vi "Init Command.vi"(5 "Sequencer":refnum<class "MessageQ.lvclass">, 6 "Variables":refnum<class "Variables.lvclass">, 7 "VolatusAPI":refnum<class "VolatusAPI.lvclass">, 8 "error in (no error)":refnum<class "MultiErrors.lvclass">, 10 "Command Config":refnum<class "Command Config.lvclass">, 11 "Reset Var Command in":refnum<class "Reset Var Command.lvclass">) -> (0 "error out":refnum<class "MultiErrors.lvclass">, 3 "Command":T1)   [LabVIEW 2020, in "VolatusSeq.lvlib" / "Reset Var Command.lvclass"]
uses:
  Reset Var Command.lvclass
  Reset Var Command.lvclass/Reset Var Command.ctl
  VolatusSeqConfig/Reset Var Command Config/Reset Var Command Config.lvclass
  VolatusSeqConfig/Command Type.ctl
  VolatusSeqConfig/VolatusSeqConfig.lvlib
  Volatus/MessageQ/MessageQ.lvclass
  messages/CmdDigital/Data.ctl
  messages/CmdDigital/CmdDigital.lvlib
  messages/CmdAnalog/Data.ctl
  messages/CmdAnalog/CmdAnalog.lvlib
  Send Type.ctl
  VolatusSeq.lvlib
  Command.ctl
  Variables/Variables.lvclass
  VolatusErrorUtilities/MultiErrors/MultiErrors.lvclass
  Volatus/VolatusAPI/VolatusAPI.lvclass
  VolatusSeqConfig/Command Config/Command Config.lvclass
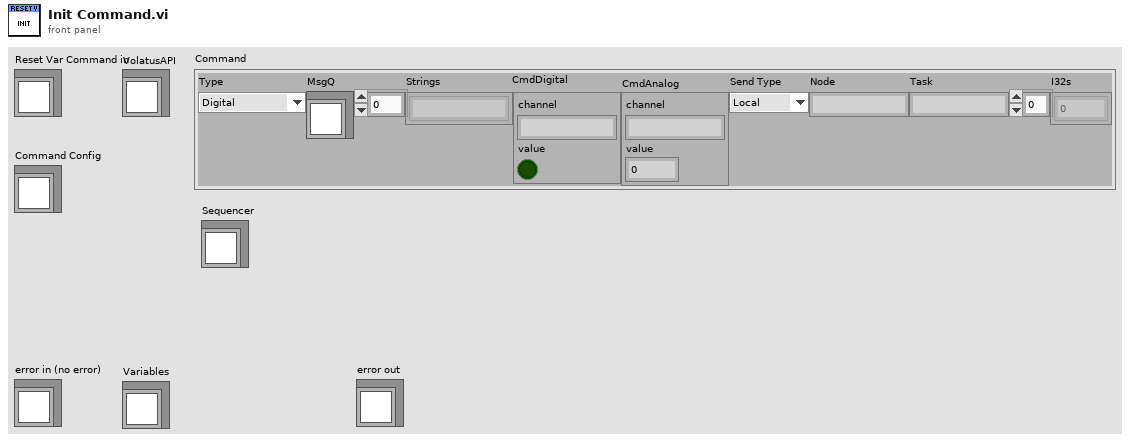
[diagram p1: front panel]
types:
  T1 = typedef "VolatusSeq.lvlib/Command.ctl" = cluster{"Type":T2, "MsgQ":refnum<class "MessageQ.lvclass">, "Strings":string[], "CmdDigital":T3, "CmdAnalog":T4, "Send Type":T5, "Node":string, "Task":string, "I32s":i32[]}
  T2 = typedef "VolatusSeqConfig.lvlib/Command Type.ctl" = enum16{"Digital", "Numeric", "Transition", "Stop", "StartLog", "StopLog", "Start", "Event", "Error", "HTTP", "ResetVar", "IncVar", "DecVar", "SaveVar", "LoadVar", "AddVar", "SubVar"}
  T3 = typedef "CmdDigital.lvlib/Data.ctl" = cluster{"channel":string, "value":bool}
  T4 = typedef "CmdAnalog.lvlib/Data.ctl" = cluster{"channel":string, "value":dbl}
  T5 = typedef "VolatusSeq.lvlib/Send Type.ctl" = enum16{"Local", "Remote"}
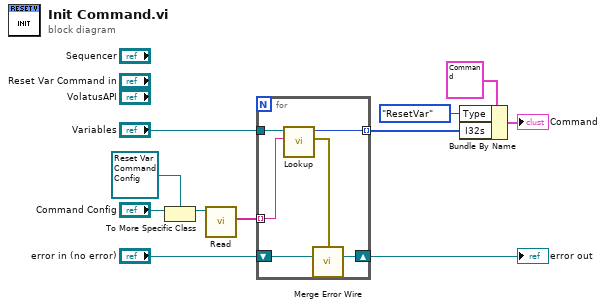
[diagram p0: block diagram]
diagram:
  n1 = To More Specific Class(target class=refnum<class "Reset Var Command Config.lvclass"> refnum ("VolatusSeqConfig.lvlib:Reset Var Command Config.lvclass"), reference="Command Config") -> (specific class reference=w9:refnum<class "Reset Var Command Config.lvclass">)  [unwired: 1 in, 1 out]
  n2 = call "Read.vi"("Reset Var Command Config in"=w9) -> ("Names"=w4:string[])  [unwired: 8 in, 2 out]
  n3 = for {
    shift-right: [w13] -> w5
    shift-left: "error in (no error)" -> [w14]
    tunnel: w4 -> [w16] mode=indexing
    tunnel: "Variables" -> [w17]
    tunnel: [w15] -> w2 mode=indexing
    n4 = call "Lookup.vi"("Name"=w16, "Variables in"=w17) -> ("error out"=w12:errorcluster, "Index"=w15:i32)  [unwired: 8 in]
    n5 = call "Merge Error Wire.vi"("error in (no error)"=w12, "MultiErrors in"=w14) -> ("MultiErrors out"=w13:refnum<class "MultiErrors.lvclass">)  [unwired: 13 in]
  }
  "error out" <- w5
  n6 = Bundle By Name(cluster=T1 {"Type"=enum."Digital", "MsgQ"=refnum, "Strings"=[], "CmdDigital"={"channel"="", "value"=FALSE}, "CmdAnalog"={"channel"="", "value"=0.0}, "Send Type"=enum."Local", "Node"="", "Task"="", "I32s"=[]} ("Command"), "Type"=Command_Type."ResetVar", "I32s"=w2) -> (→"Command":T1)
